vi "2-Byte Mono-Packed to U16.vi"(0 "2-Byte Mono Data":u8[](array[numeric]) format="%08b", 1 "Image Size":T1, 2 "Bits":i32) -> (3 "U16 Pixels":u16[][](array[numeric]) format="%04x")   [LabVIEW 2020, in "Buffer.lvclass"]
uses:
  Buffer.lvclass
  Image Size.ctl
  Buffer.lvclass/Buffer.ctl
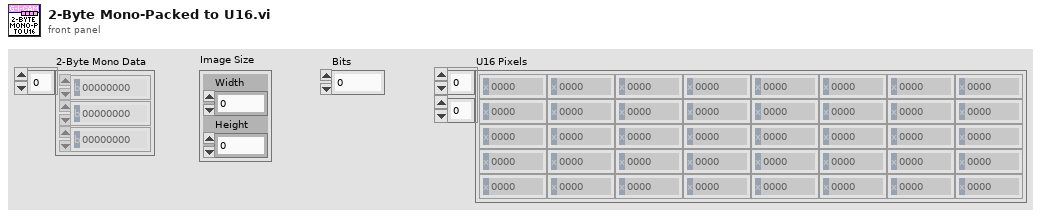
[diagram p1: front panel]
types:
  T1 = typedef "Buffer.lvclass/Image Size.ctl" = cluster{"Width":u16, "Height":u16}
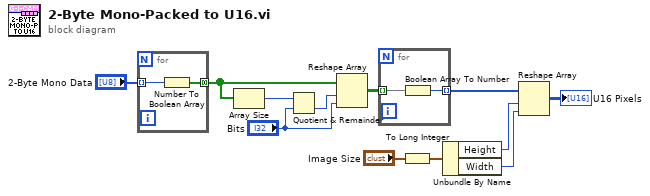
[diagram p0: block diagram]
diagram:
  n1 = for {
    tunnel: "2-Byte Mono Data" -> [w14] mode=indexing
    tunnel: [w13] -> w11 mode=concatenating
    n2 = Number To Boolean Array(number=w14) -> (Boolean array=w13:bool[])
  }
  n3 = Array Size(array=w11) -> (size(s)=w10:i32)
  n4 = Quotient & Remainder(x=w10, y="Bits") -> (floor(x/y)=w9:i32)  [unwired: 1 out]
  n5 = Reshape Array(w11, w9, "Bits") -> (w8:bool[][])
  n6 = for {
    tunnel: w8 -> [w16] mode=indexing
    tunnel: [w15] -> w7 mode=indexing
    n7 = Boolean Array To Number(Boolean array=w16) -> (number=w15:u16)
  }
  n8 = To Long Integer(number="Image Size") -> (32bit integer=w3:cluster{"Width":i32, "Height":i32})
  n9 = Unbundle By Name(w3) -> ("Height"=w1:i32, "Width"=w2:i32)
  n10 = Reshape Array(w7, w1, w2) -> (→"U16 Pixels":u16[][])
